vi "SIM limit new stepsize.vi"(6 "min step size":dbl, 7 "current timestep base":dbl, 8 "error":errorcluster, 9 "proposed step time":dbl, 10 "proposed step size":dbl, 11 "step size":dbl) -> (0 "error out":errorcluster, 2 "proposed step size":dbl, 3 "step size":dbl)   [LabVIEW 2020]
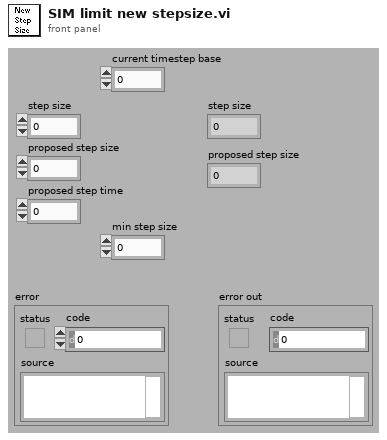
[diagram p1: front panel]
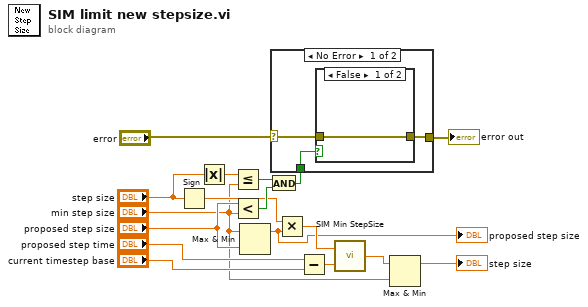
[diagram p0: block diagram]
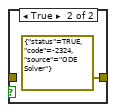
[diagram p2: hidden frame]
diagram:
  n1 = Sign(1:"step size") -> (0:w13:dbl)
  n2 = Absolute Value(x="step size") -> (abs(x)=w14:dbl)
  n3 = Less Or Equal?(x=w14, y="min step size") -> (x <= y?=w16:bool)
  n4 = Less?(x="proposed step size", y="min step size") -> (x < y?=w15:bool)
  n5 = Max & Min(x="min step size", y="proposed step size") -> (max(x,y)=w11:dbl)  [unwired: 1 out]
  "proposed step size" <- w11
  n6 = And(x=w16, y=w15) -> (x .and. y?=w6:bool)
  n7 = case shown="No Error" "error" {
    selector: "error" -> [w19 w23]
    tunnel: w6 -> [w20 _]
    tunnel: [w18 w23] -> w5
    frame No Error {
      n8 = case shown="False" w20 {
        tunnel: [w21 errorcluster {"status"=TRUE, "code"=-2324, "source"="ODE Solver"} ("error")] -> w18
        tunnel: w19 -> [w21 _]
        frame False {
        }
        frame True {
        }
      }
    }
    frame Error {
    }
  }
  "error out" <- w5
  n9 = Multiply(x=w13, y=w11) -> (x*y=w12:dbl)
  n10 = Subtract(x="proposed step time", y="current timestep base") -> (x-y=w17:dbl)
  n11 = call "SIM Min StepSize.vi"("step size 2"=w17, "step size 1"=w12) -> ("min step size"=w3:dbl)
  n12 = Max & Min(x=w3, y="min step size") -> (max(x,y)=→"step size":dbl)  [unwired: 1 out]
